vi "SeCrTS-DD NS Data Storage.vi"(8 "error in":errorcluster, 9 "AI_V_Data P\nAI_C_Data P\nAO_Data P\nDO_Data P\nACC_Data P\nTC Data P\nDrive_A_C \nDrive_A_D\nAI_C_Data S\nDO_Data S":refnum<queue>[](array[refnum]), 10 "Data in":string, 11 "DI P\nDI S":refnum<queue>[](array[refnum])) -> (0 "error out":errorcluster)   [LabVIEW 2022 SP3]
panel:
  out "overflow? 5":bool
  out "overflow? 3":bool
  out "overflow? 2":bool
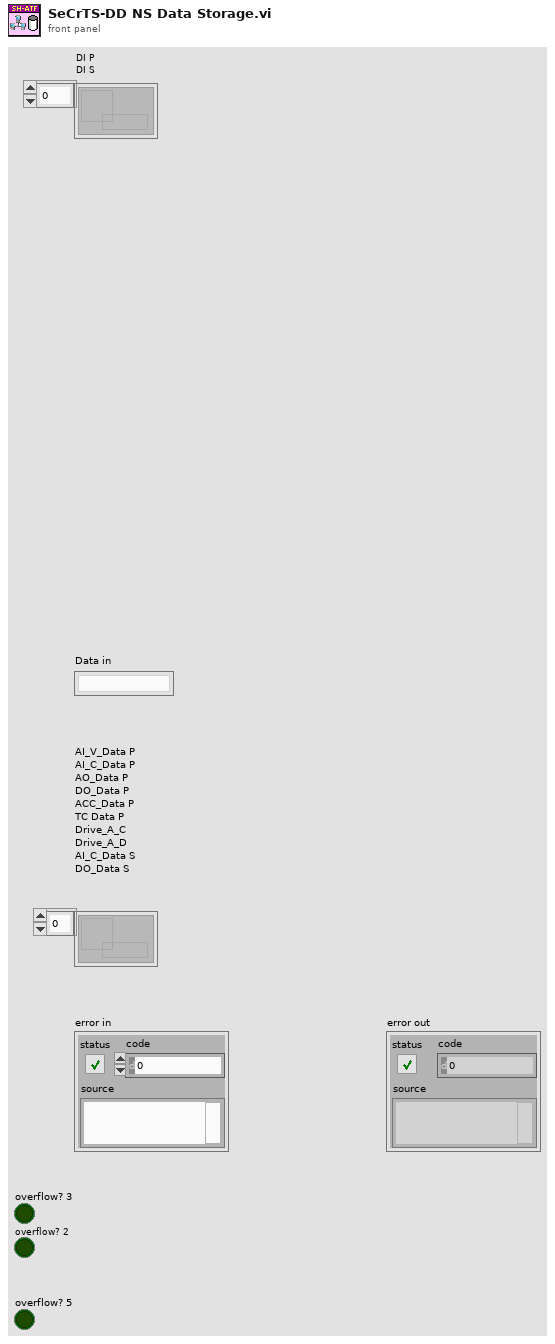
[diagram p1: front panel]
types:
  T1 = cluster{"AI_V_Data":waveform(dbl)[][], "DO_Data":waveform(dbl)[][], "DI_Data":digitalwaveform[][]}
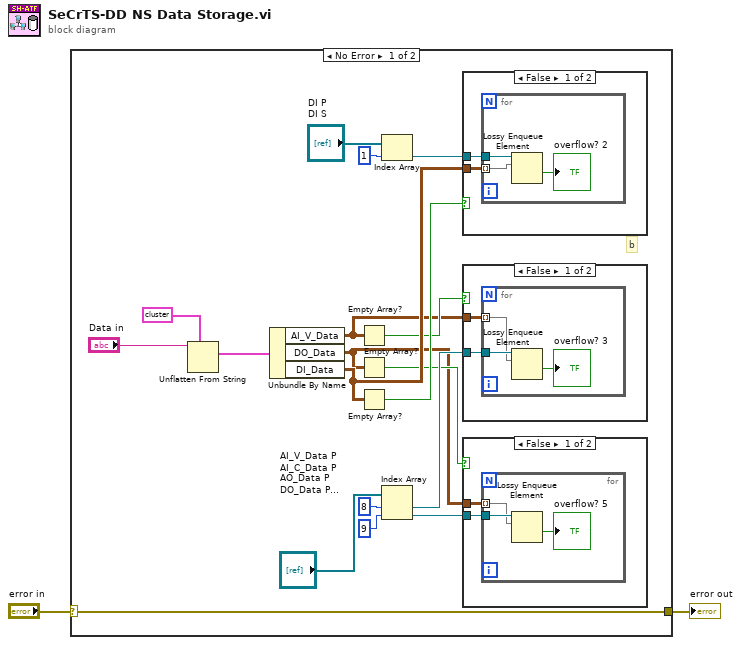
[diagram p0: block diagram]
diagram:
  n1 = case shown="No Error" "error in" {
    selector: "error in" -> [w3 w36]
    tunnel: [w3 w36] -> w1
    frame No Error {
      # "b"
      n2 = Unflatten From String(type=T1 data[100104B] ("data out"), binary string="Data in") -> (value=w4:T1)  [unwired: 3 in, 2 out]
      n3 = Unbundle By Name(w4) -> ("AI_V_Data"=w12:waveform(dbl)[][], "DO_Data"=w10:waveform(dbl)[][], "DI_Data"=w14:digitalwaveform[][])
      n4 = Empty Array?(array=w12) -> (empty?=w13:bool)
      n5 = Empty Array?(array=w10) -> (empty?=w11:bool)
      n6 = Empty Array?(array=w14) -> (empty?=w15:bool)
      n7 = Index Array(array="DI P\nDI S", index=1) -> (element=w6:refnum<queue>)
      n8 = Index Array(array="AI_V_Data P\nAI_C_Data P\nAO_Data P\nDO_Data P\nACC_Data P\nTC Data P\nDrive_A_C \nDrive_A_D\nAI_C_Data S\nDO_Data S", index #1=8 ("index"), index #2=9 ("index")) -> (element #1=w17:refnum<queue>, element #2=w8:refnum<queue>)
      n9 = case shown="False" w15 {
        tunnel: w14 -> [w32 _]
        tunnel: w6 -> [w31 _]
        frame False {
          n10 = for {
            tunnel: w32 -> [w33] mode=indexing
            tunnel: w31 -> [w35]
            n11 = Lossy Enqueue Element(queue=w35, element=w33) -> (overflow?=→"overflow? 2":bool)  [unwired: 1 in, 3 out]
          }
        }
        frame True {
        }
      }
      n12 = case shown="False" w13 {
        tunnel: w12 -> [w27 _]
        tunnel: w17 -> [w26 _]
        frame False {
          n13 = for {
            tunnel: w27 -> [w28] mode=indexing
            tunnel: w26 -> [w30]
            n14 = Lossy Enqueue Element(queue=w30, element=w28) -> (overflow?=→"overflow? 3":bool)  [unwired: 1 in, 3 out]
          }
        }
        frame True {
        }
      }
      n15 = case shown="False" w11 {
        tunnel: w10 -> [w22 _]
        tunnel: w8 -> [w21 _]
        frame False {
          n16 = for {
            tunnel: w22 -> [w23] mode=indexing
            tunnel: w21 -> [w25]
            n17 = Lossy Enqueue Element(queue=w25, element=w23) -> (overflow?=→"overflow? 5":bool)  [unwired: 1 in, 3 out]
          }
        }
        frame True {
        }
      }
    }
    frame Error {
    }
  }
  "error out" <- w1
